vi "record_position.vi"(8 "错误输入（无错误）":errorcluster) -> (0 "错误输出":errorcluster)   [LabVIEW 2013]
uses:
  <vilib>/Utility/file.llb/Write To Spreadsheet File (DBL).vi
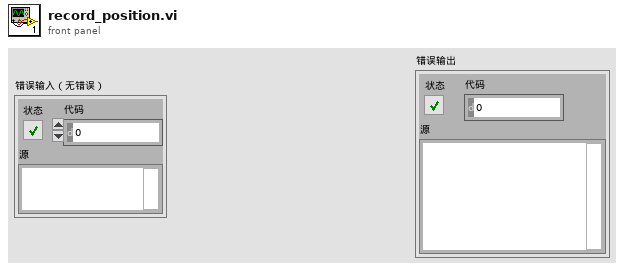
[diagram p1: front panel]
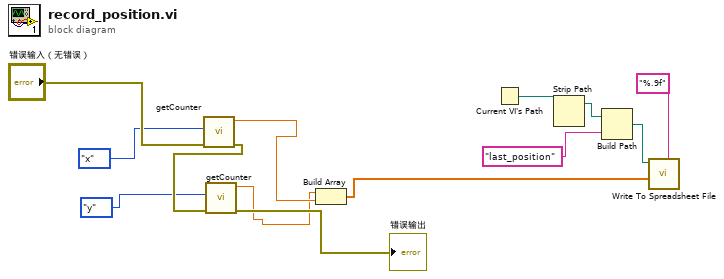
[diagram p0: block diagram]
diagram:
  n1 = call "getCounter.vi"("错误输入（无错误）"="错误输入（无错误）", "channel"=enum16{"x", "y"}."x" ("axie")) -> ("错误输出"=w13:errorcluster, "result"=w8:dbl)  [unwired: 8 in]
  n2 = call "getCounter.vi"("错误输入（无错误）"=w13, "channel"=enum16{"x", "y"}."y" ("axie")) -> ("错误输出"=→"错误输出":errorcluster, "result"=w7:dbl)  [unwired: 8 in]
  n3 = Build Array(w7, w8) -> (w1:dbl[])
  n4 = Current VI's Path() -> (path=w4:path)
  n5 = Strip Path(path=w4) -> (stripped path=w3:path)  [unwired: 1 out]
  n6 = Build Path(base path=w3, name or relative path="last_position") -> (appended path=w5:path)
  n7 = call-poly <vilib>:"Write To Spreadsheet File.vi"("format (%.3f)"="%.9f", "1D data"=w1, "file path (dialog if empty)"=w5) -> ()  [unwired: 5 in, 1 out]
